vi "Mapping Countdown.vi"(6 "Execution Times (s)":dbl[](array[numeric]), 7 "Forward?":bool, 8 "Drive Velocity":dbl=10.0 caption="Velocity (V/s)" min=10.0 max=160.0 step=0.1 format="%.1f", 9 "Mapping Spectra Settings":T1={"Integration Time"=10.0, "Repetitions"=10, "Mapping Spectra"=TRUE} {"Repetitions" min=1 max=100 step=1; "Integration Time" min=0.5 max=6000.0 step=1.0 format="%.1f"}, 10 "Drive New Abs. Positions":T2={"Drive X Set"=10.0, "Drive Y Set"=10.0, "Drive Z Set"=10.0} {"Drive X Set" min=10.0 max=160.0 step=0.1 format="%.1f"; "Drive Z Set" min=10.0 max=160.0 step=0.1 format="%.1f"; "Drive Y Set" min=10.0 max=160.0 step=0.1 format="%.1f"}, 11 "Mapping Drive Parameters":T3={"X Start Position"=10.0, "X Stop Position"=10.0, "Y Start Position"=10.0, "Y Stop Position"=10.0, "Step Size"=10.0} {"Step Size" min=0.1 max=30.0 step=0.1 format="%.1f"; "Y Stop Position" min=0.0 max=30.0 step=0.1 format="%.1f"; "Y Start Position" min=0.0 max=30.0 step=0.1 format="%.1f"; "X Stop Position" min=0.0 max=30.0 step=0.1 format="%.1f"; "X Start Position" min=0.0 max=30.0 step=0.1 format="%.1f"}) -> (2 "Progress":i16, 3 "Time String":string)   [LabVIEW 2010]
uses:
  TypeDefs/Mapping Drive Params.ctl
  ESA-C/TypeDefs/ESA-C Set Positions.ctl
  TypeDefs/Mapping Spectra Params.ctl
  <vilib>/Analysis/NI_AALBase.lvlib
panel:
  out "Step Time (s)":dbl
  out "Left Time (s)":dbl
  out "Left Steps":dbl
  out "Ready Steps":dbl
  out "Ready Cols":dbl
  out "Ready Rows":dbl
  out "Total Steps":dbl
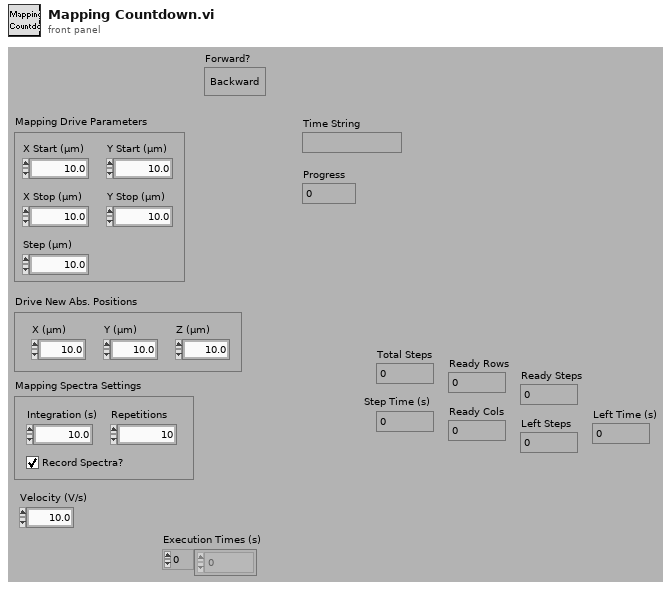
[diagram p1: front panel]
types:
  T1 = typedef "Mapping Spectra Params.ctl" = cluster{"Integration Time":dbl, "Repetitions":u16, "Mapping Spectra":bool}
  T2 = typedef "ESA-C Set Positions.ctl" = cluster{"Drive X Set":dbl, "Drive Y Set":dbl, "Drive Z Set":dbl}
  T3 = typedef "Mapping Drive Params.ctl" = cluster{"X Start Position":dbl, "X Stop Position":dbl, "Y Start Position":dbl, "Y Stop Position":dbl, "Step Size":dbl}
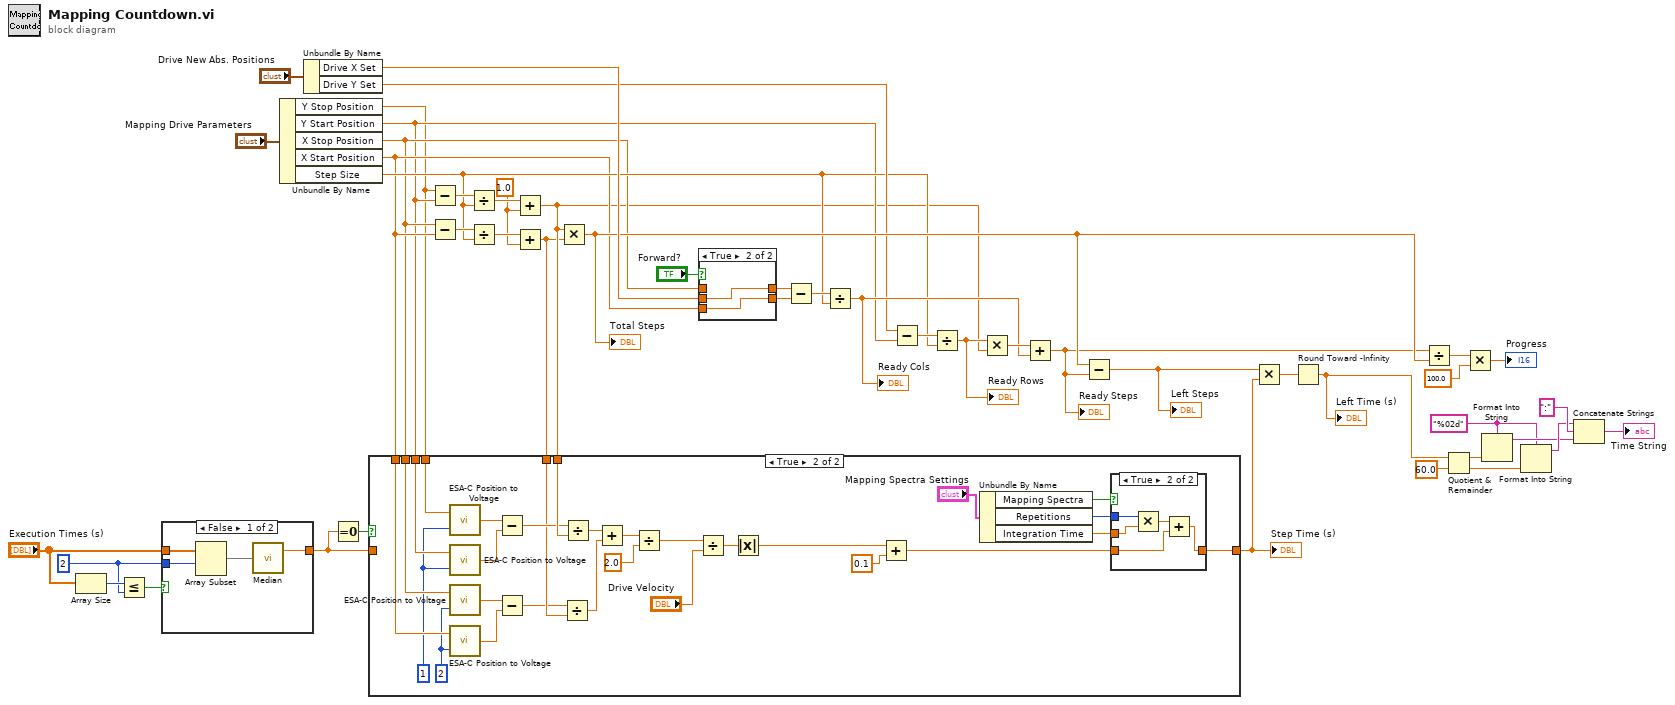
[diagram p0: block diagram]
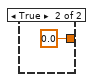
[diagram p2: hidden frame]
diagram:
  w3 = 2 ("index")
  w24 = 1.0 ("y")
  w42 = "%02d" ("Format-String")
  n1 = Array Size(array="Execution Times (s)") -> (size(s)=w6:i32)
  n2 = Less Or Equal?(x=w6, y=w3) -> (x <= y?=w5:bool)
  n3 = case shown="False" w5 {
    tunnel: "Execution Times (s)" -> [w50 _]
    tunnel: w3 -> [w49 _]
    tunnel: [w48 0.0 ("mean")] -> w2
    frame False {
      n4 = Array Subset(array=w50, index=w49) -> (w51:dbl[])  [unwired: 1 in]
      n5 = call <vilib>:"Median.vi"("X"=w51) -> ("median"=w48:dbl)  [unwired: 1 out]
    }
    frame True {
    }
  }
  n6 = Unbundle By Name("Mapping Drive Parameters") -> ("Y Stop Position"=w10:dbl, "Y Start Position"=w11:dbl, "X Stop Position"=w12:dbl, "X Start Position"=w13:dbl, "Step Size"=w14:dbl)
  n7 = Unbundle By Name("Drive New Abs. Positions") -> ("Drive X Set"=w32:dbl, "Drive Y Set"=w15:dbl)
  n8 = Equal To 0?(x=w2) -> (x = 0?=w7:bool)
  n9 = Subtract(x=w10, y=w11) -> (x-y=w29:dbl)
  n10 = Subtract(x=w12, y=w13) -> (x-y=w28:dbl)
  n11 = Divide(x=w29, y=w14) -> (x/y=w26:dbl)
  n12 = Divide(x=w28, y=w14) -> (x/y=w27:dbl)
  n13 = Add(x=w26, y=w24) -> (x+y=w9:dbl)
  n14 = Add(x=w27, y=w24) -> (x+y=w8:dbl)
  n15 = case shown="True" w7 {
    tunnel: [w53 w77] -> w1
    tunnel: w13 -> [_ w75]
    tunnel: w12 -> [_ w74]
    tunnel: w11 -> [_ w73]
    tunnel: w10 -> [_ w72]
    tunnel: w9 -> [_ w65]
    tunnel: w8 -> [_ w63]
    tunnel: w2 -> [w53 _]
    frame False {
    }
    frame True {
      w70 = 2 ("Axis")
      w71 = 1 ("Axis")
      n16 = call "ESA-C Position to Voltage.vi"("Axis"=w71, "Position (µm)"=w72) -> ("Voltage (V)"=w69:dbl)
      n17 = call "ESA-C Position to Voltage.vi"("Axis"=w71, "Position (µm)"=w73) -> ("Voltage (V)"=w68:dbl)
      n18 = call "ESA-C Position to Voltage.vi"("Axis"=w70, "Position (µm)"=w74) -> ("Voltage (V)"=w67:dbl)
      n19 = call "ESA-C Position to Voltage.vi"("Axis"=w70, "Position (µm)"=w75) -> ("Voltage (V)"=w66:dbl)
      n20 = Subtract(x=w69, y=w68) -> (x-y=w64:dbl)
      n21 = Subtract(x=w67, y=w66) -> (x-y=w62:dbl)
      n22 = Divide(x=w62, y=w63) -> (x/y=w60:dbl)
      n23 = Divide(x=w64, y=w65) -> (x/y=w61:dbl)
      n24 = Add(x=w61, y=w60) -> (x+y=w59:dbl)
      n25 = Divide(x=w59, y=2.0) -> (x/y=w57:dbl)
      n26 = Divide(x=w57, y="Drive Velocity") -> (x/y=w55:dbl)
      n27 = Absolute Value(x=w55) -> (abs(x)=w54:dbl)
      n28 = Add(x=w54, y=0.1) -> (x+y=w76:dbl)
      n29 = Unbundle By Name("Mapping Spectra Settings") -> ("Mapping Spectra"=w80:bool, "Repetitions"=w79:u16, "Integration Time"=w78:dbl)
      n30 = case shown="True" w80 {
        tunnel: w79 -> [_ w88]
        tunnel: w78 -> [_ w87]
        tunnel: w76 -> [w83 w85]
        tunnel: [w83 w84] -> w77
        frame False {
        }
        frame True {
          n31 = Multiply(x=w88, y=w87) -> (x*y=w86:dbl)
          n32 = Add(x=w86, y=w85) -> (x+y=w84:dbl)
        }
      }
    }
  }
  "Step Time (s)" <- w1
  n33 = Multiply(x=w9, y=w8) -> (x*y=w19:dbl)
  "Total Steps" <- w19
  n34 = case shown="True" "Forward?" {
    tunnel: w32 -> [w90 w92]
    tunnel: w13 -> [_ w91]
    tunnel: w12 -> [w89 _]
    tunnel: [w90 w91] -> w31
    tunnel: [w89 w92] -> w30
    frame False {
    }
    frame True {
    }
  }
  n35 = Subtract(x=w30, y=w31) -> (x-y=w23:dbl)
  n36 = Divide(x=w23, y=w14) -> (x/y=w20:dbl)
  "Ready Cols" <- w20
  n37 = Subtract(x=w15, y=w11) -> (x-y=w25:dbl)
  n38 = Divide(x=w25, y=w14) -> (x/y=w22:dbl)
  "Ready Rows" <- w22
  n39 = Multiply(x=w22, y=w9) -> (x*y=w21:dbl)
  n40 = Add(x=w21, y=w20) -> (x+y=w18:dbl)
  "Ready Steps" <- w18
  n41 = Subtract(x=w19, y=w18) -> (x-y=w17:dbl)
  "Left Steps" <- w17
  n42 = Multiply(x=w17, y=w1) -> (x*y=w36:dbl)
  n43 = Round Toward -Infinity(1:w36) -> (0:w39:dbl)
  "Left Time (s)" <- w39
  n44 = Divide(x=w18, y=w19) -> (x/y=w16:dbl)
  n45 = Quotient & Remainder(x=w39, y=60.0) -> (x-y*floor(x/y)=w41:dbl, floor(x/y)=w40:dbl)
  n46 = Multiply(x=w16, y=100.0) -> (x*y=→"Progress":dbl)
  n47 = Format Into String(format string=w42, w41) -> (resulting string=w43:string)  [unwired: 2 in, 1 out]
  n48 = Format Into String(format string=w42, w40) -> (resulting string=w44:string)  [unwired: 2 in, 1 out]
  n49 = Concatenate Strings(w44, ":" ("String"), w43) -> (→"Time String":string)
